vi "Scroll-Hmove.vi"(8 "error in (no error)":errorcluster, 9 "New coordinate":T1, 11 "Gviewer in":refnum<class "Gviewer.lvclass">) -> (0 "error out":errorcluster, 3 "Gviewer out":refnum<class "Gviewer.lvclass">)   [LabVIEW 2020, in "Gviewer.lvclass"]
doc: "Andre Koelewijn, 14 feb 2021\n\nThis VI perform the actual horizontal move in respect to the position where the mouse was clicked."
uses:
  Gviewer.lvclass
  <vilib>/Utility/miscctls.llb/LVPoint32TypeDef.ctl
  Gviewer.lvclass/Gviewer.ctl
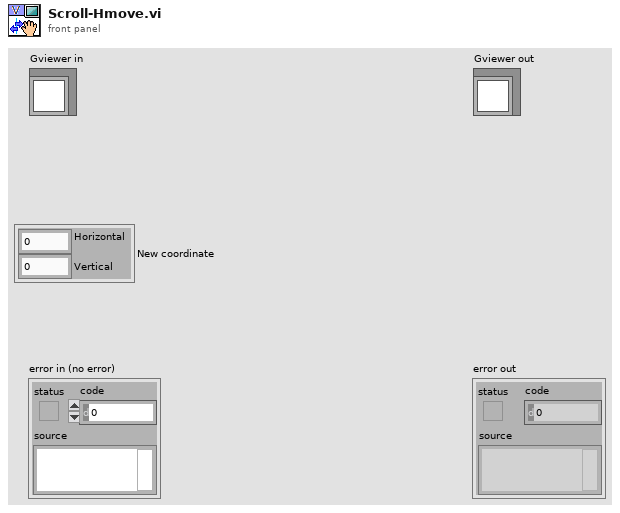
[diagram p1: front panel]
types:
  T1 = typedef "LVPoint32TypeDef.ctl" = cluster{"Horizontal":i32, "Vertical":i32}
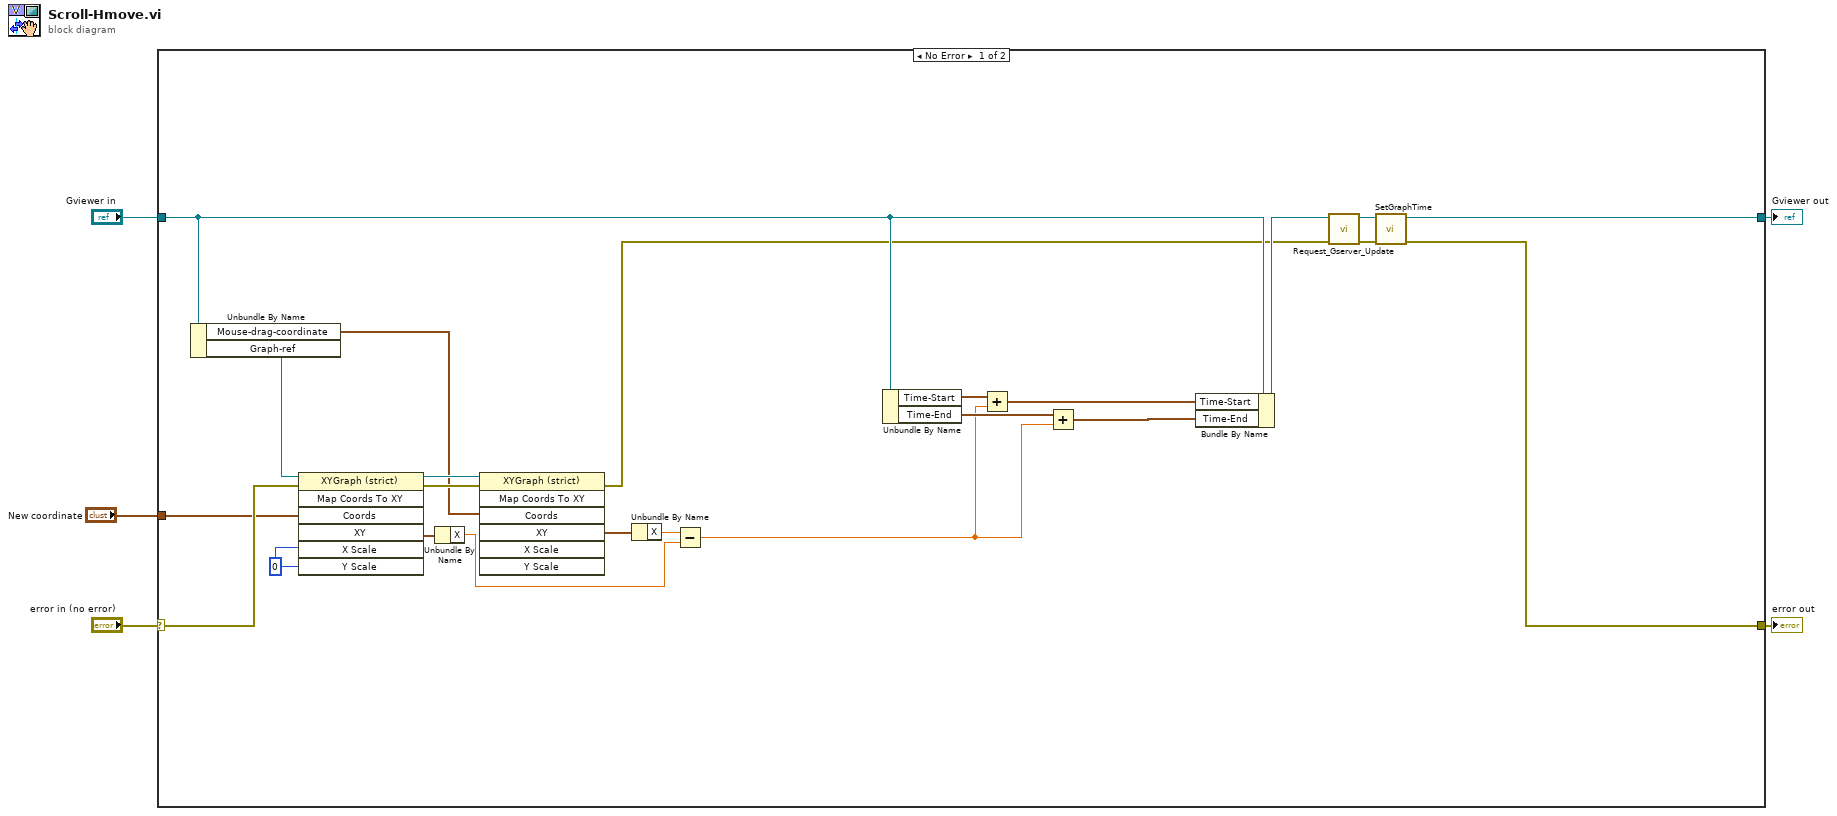
[diagram p0: block diagram]
diagram:
  n1 = case shown="No Error" "error in (no error)" {
    selector: "error in (no error)" -> [w26 w30]
    tunnel: [w11 w30] -> w4
    tunnel: [w14 w29] -> w2
    tunnel: "Gviewer in" -> [w13 w29]
    tunnel: "New coordinate" -> [w25 _]
    frame No Error {
      w28 = 0 ("Y Scale")
      n2 = Unbundle By Name(w13) -> ("Mouse-drag-coordinate"=w21:T1, "Graph-ref"=w20:refnum<vi>)
      n3 = invoke class="XYGraph (strict)" method="Map Coords To XY"(reference=w20, error in=w26, "Coords"=w25, "X Scale"=w28, "Y Scale"=w28) -> (reference out=w22:refnum<vi>, error out=w23:errorcluster, "XY"=w27:cluster{"X":dbl, "Y":dbl})  [unwired: 2 in, 4 out]
      n4 = Unbundle By Name(w27) -> ("X"=w18:dbl)
      n5 = invoke class="XYGraph (strict)" method="Map Coords To XY"(reference=w22, error in=w23, "Coords"=w21) -> (error out=w12:errorcluster, "XY"=w24:cluster{"X":dbl, "Y":dbl})  [unwired: 4 in, 5 out]
      n6 = Unbundle By Name(w24) -> ("X"=w19:dbl)
      n7 = Subtract(x=w19, y=w18) -> (x-y=w7:dbl)
      n8 = Unbundle By Name(w13) -> ("Time-Start"=w10:timestamp, "Time-End"=w9:timestamp)
      n9 = Add(x=w10, y=w7) -> (x+y=w8:timestamp)
      n10 = Add(x=w9, y=w7) -> (x+y=w6:timestamp)
      n11 = Bundle By Name(cluster=w13, "Time-Start"=w8, "Time-End"=w6) -> (w17:refnum<class "Gviewer.lvclass">)
      n12 = call "Request_Gserver_Update.vi"("error in (no error)"=w12, "Gviewer in"=w17) -> ("error out"=w15:errorcluster, "Gviewer out"=w16:refnum<class "Gviewer.lvclass">)  [unwired: 8 in]
      n13 = call "SetGraphTime.vi"("error in (no error)"=w15, "Gviewer in"=w16) -> ("error out"=w11:errorcluster, "Gviewer out"=w14:refnum<class "Gviewer.lvclass">)  [unwired: 8 in]
    }
    frame Error {
    }
  }
  "error out" <- w4
  "Gviewer out" <- w2
